vi "LoopBackResultTx.vi"(8 "error in (no error)":errorcluster, 11 "map":map{string, string}(c390)) -> (0 "error out":errorcluster, 2 "status":string)   [LabVIEW 2021]
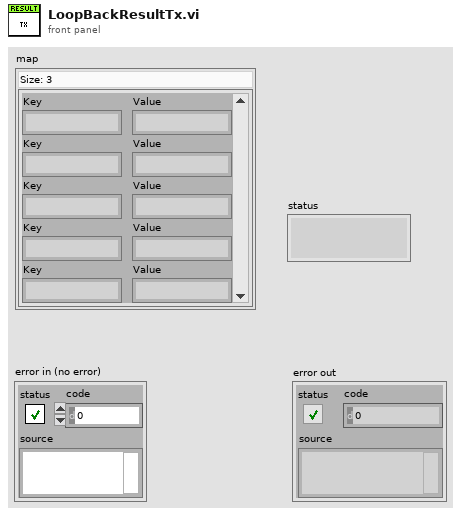
[diagram p1: front panel]
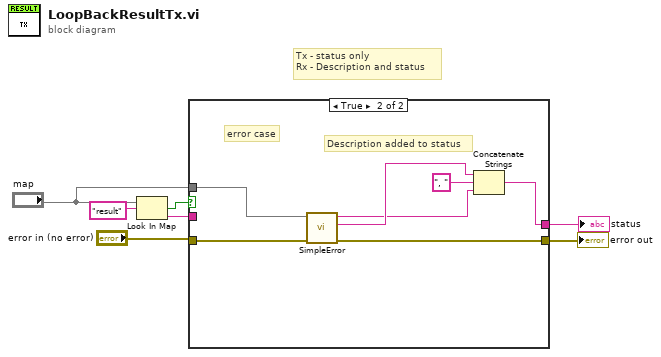
[diagram p0: block diagram]
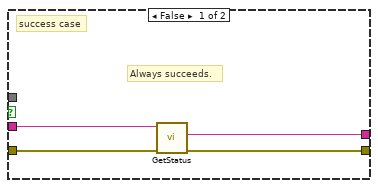
[diagram p2: hidden frame]
diagram:
  # "Tx - status only\nRx - Description and status"
  n1 = Look In Map(map="map", key="result") -> (key not found?=w5:bool, value=w6:string)  [unwired: 1 in]
  n2 = case shown="True" w5 {
    tunnel: w6 -> [w11 _]
    tunnel: "error in (no error)" -> [w10 w18]
    tunnel: [w9 w17] -> w3
    tunnel: "map" -> [_ w16]
    tunnel: [w8 w12] -> w1
    frame False {
      # "Always succeeds."
      # "success case"
      n3 = call "GetStatus.vi"("error in (no error)"=w10, "Value"=w11) -> ("error out"=w9:errorcluster, "status"=w8:string)  [unwired: 7 in, 1 out]
    }
    frame True {
      # "Description added to status"
      # "error case"
      n4 = call "SimpleError.vi"("error in (no error)"=w18, "map"=w16) -> ("error out"=w17:errorcluster, "status"=w14:string, "description"=w13:string)  [unwired: 7 in]
      n5 = Concatenate Strings(w14, ", " ("string"), w13) -> (w12:string)
    }
  }
  "error out" <- w3
  "status" <- w1
